vi "RoomReportDataToGraph.vi"(8 "Error In":errorcluster, 10 "RoomReport":T2) -> (0 "Error Out":errorcluster, 2 "RoomGraphs":T1 {"NurseAvgFulfillTime(s)" scale=0.0..100.0; "DrAvgFulfillTime(s)" scale=0.0..200.0; "#NurseAlarms" scale=0.0..10.0; "#Patients" scale=0.0..10.0; "#DrAlarms" scale=0.0..10.0; "AvgStayPerRoom(s)" scale=0.0..10.0})   [LabVIEW 2015]
uses:
  TypeDef/RoomReport.ctl
  TypeDef/RoomReportGraphs.ctl
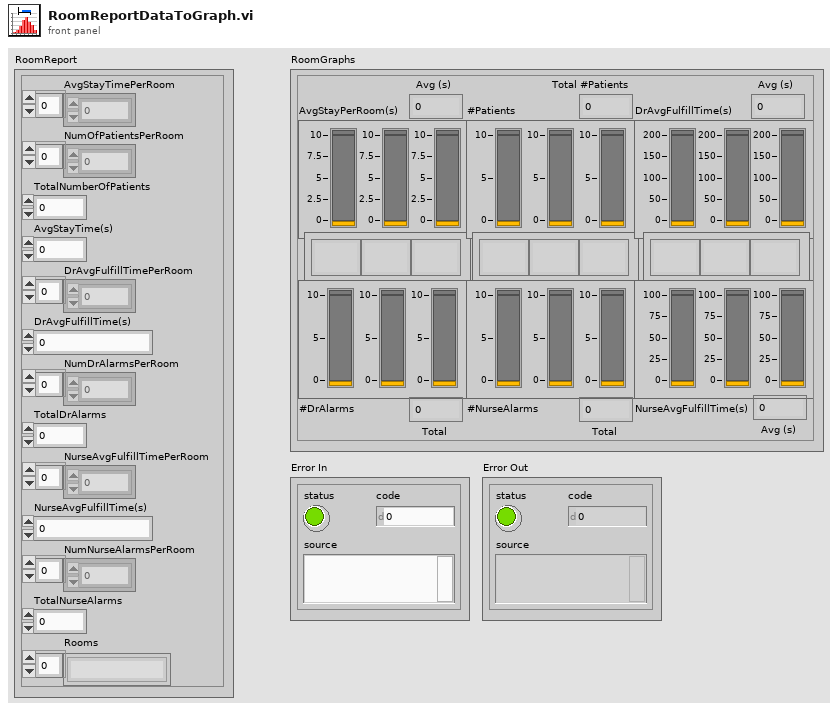
[diagram p1: front panel]
types:
  T1 = typedef "RoomReportGraphs.ctl" = cluster{"AvgStay (s)":dbl, "AvgStayPerRoom(s)":dbl[], "Total #Patients":i32, "#Patients":i32[], "TotalDrAvgFulfillTime(s)":dbl, "DrAvgFulfillTime(s)":dbl[], "#DrAlarms":i32[], "TotalDrAlarms":i32, "#NurseAlarms":i32[], "TotalNurseAlarms":i32, "NurseAvgFulfillTime(s)":dbl[], "TotalNurseAvgFulfillTime(s)":dbl, "RoomNumArr1":string[], "RoomNumArr2":string[], "RoomNumArr3":string[]}
  T2 = typedef "RoomReport.ctl" = cluster{"AvgStayTimePerRoom":dbl[], "NumOfPatientsPerRoom":i32[], "TotalNumberOfPatients":i32, "AvgStayTime(s)":dbl, "DrAvgFulfillTimePerRoom":dbl[], "DrAvgFulfillTime(s)":dbl, "NumDrAlarmsPerRoom":i32[], "TotalDrAlarms":i32, "NurseAvgFulfillTimePerRoom":dbl[], "NurseAvgFulfillTime(s)":dbl, "NumNurseAlarmsPerRoom":i32[], "TotalNurseAlarms":i32, "Rooms":string[]}
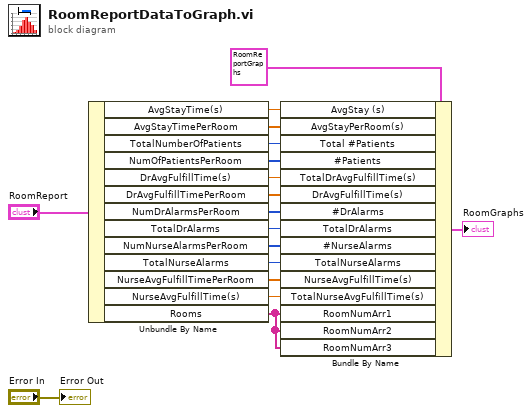
[diagram p0: block diagram]
diagram:
  n1 = Unbundle By Name("RoomReport") -> ("AvgStayTime(s)"=w15:dbl, "AvgStayTimePerRoom"=w14:dbl[], "TotalNumberOfPatients"=w13:i32, "NumOfPatientsPerRoom"=w12:i32[], "DrAvgFulfillTime(s)"=w11:dbl, "DrAvgFulfillTimePerRoom"=w10:dbl[], "NumDrAlarmsPerRoom"=w8:i32[], "TotalDrAlarms"=w7:i32, "NumNurseAlarmsPerRoom"=w6:i32[], "TotalNurseAlarms"=w5:i32, "NurseAvgFulfillTimePerRoom"=w4:dbl[], "NurseAvgFulfillTime(s)"=w3:dbl, "Rooms"=w2:string[])
  n2 = Bundle By Name(cluster=T1 {"AvgStay (s)"=0.0, "AvgStayPerRoom(s)"=[], "Total #Patients"=0, "#Patients"=[], "TotalDrAvgFulfillTime(s)"=0.0, "DrAvgFulfillTime(s)"=[], "#DrAlarms"=[], "TotalDrAlarms"=0, "#NurseAlarms"=[], "TotalNurseAlarms"=0, "NurseAvgFulfillTime(s)"=[], "TotalNurseAvgFulfillTime(s)"=0.0, "RoomNumArr1"=[], "RoomNumArr2"=[], "RoomNumArr3"=[]} ("RoomGraphs"), "AvgStay (s)"=w15, "AvgStayPerRoom(s)"=w14, "Total #Patients"=w13, "#Patients"=w12, "TotalDrAvgFulfillTime(s)"=w11, "DrAvgFulfillTime(s)"=w10, "#DrAlarms"=w8, "TotalDrAlarms"=w7, "#NurseAlarms"=w6, "TotalNurseAlarms"=w5, "NurseAvgFulfillTime(s)"=w4, "TotalNurseAvgFulfillTime(s)"=w3, "RoomNumArr1"=w2, "RoomNumArr2"=w2, "RoomNumArr3"=w2) -> (→"RoomGraphs":T1)
  "Error Out" <- "Error In"
